vi "GV_LegendVisible.vi"(8 "error in (no error)":errorcluster, 11 "Gviewer in":refnum<class "Gviewer.lvclass">) -> (0 "error out":errorcluster, 1 "Visible?":bool, 3 "Gviewer out":refnum<class "Gviewer.lvclass">)   [LabVIEW 2020, in "Sgraph_lib_V1.lvlib" / "Gviewer.lvclass"]
doc: "Andre Koelewijn, 24 April 2021,\n\nShow/Hide Legend"
uses:
  Gviewer.lvclass
  Gviewer.lvclass/Gviewer.ctl
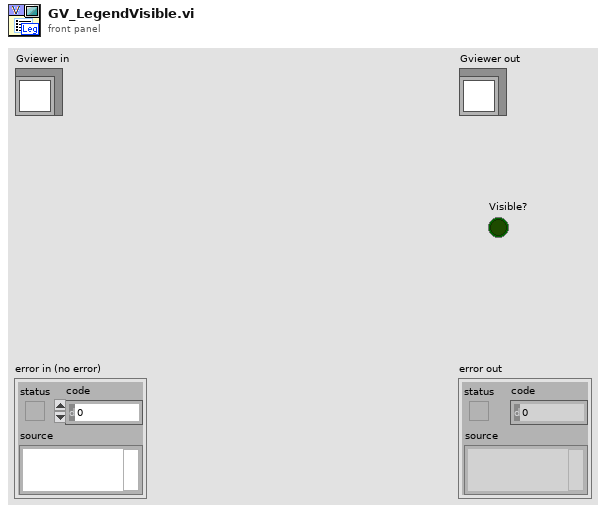
[diagram p1: front panel]
types:
  T1 = typedef "LVPositionTypeDef.ctl" = cluster{"Left":i32, "Top":i32}
  T2 = typedef "LVBoundsTypeDef.ctl" = cluster{"Width":u32, "Height":u32}
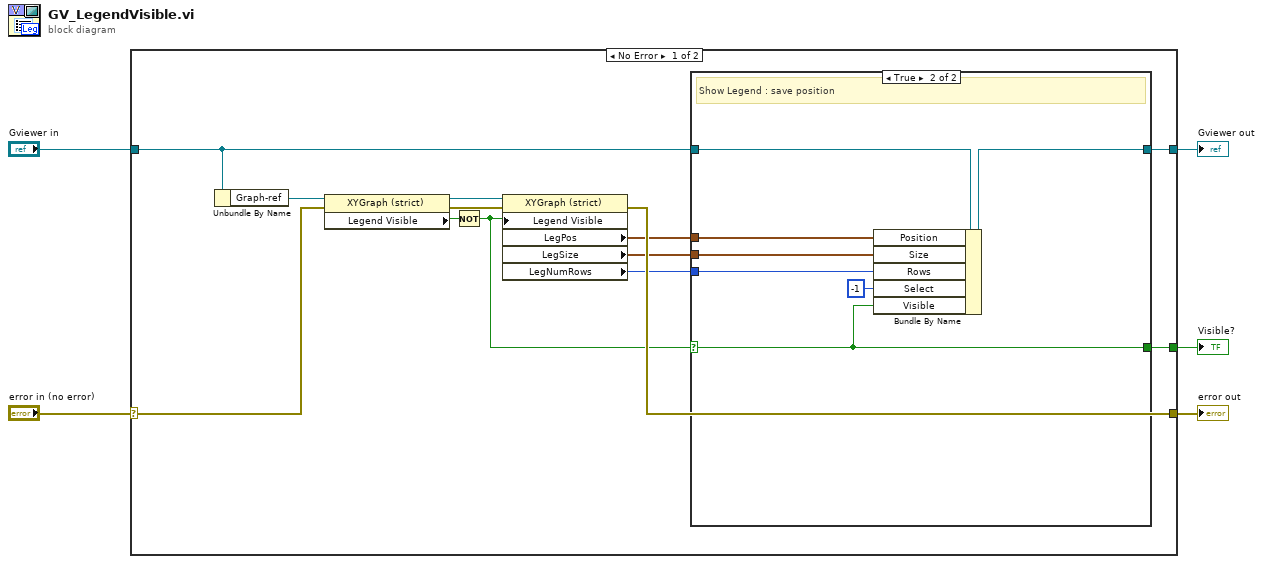
[diagram p0: block diagram]
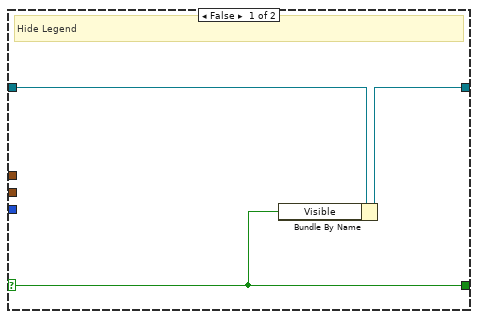
[diagram p2: hidden frame]
diagram:
  n1 = case shown="No Error" "error in (no error)" {
    selector: "error in (no error)" -> [w14 w30]
    tunnel: [w13 w30] -> w4
    tunnel: [w9 w29] -> w2
    tunnel: "Gviewer in" -> [w10 w29]
    tunnel: [w11 _] -> w1
    frame No Error {
      n2 = Unbundle By Name(w10) -> ("Graph-ref"=w15:refnum<vi>)
      n3 = property class="XYGraph (strict)"(reference=w15, error in=w14) -> (reference out=w16:refnum<vi>, error out=w17:errorcluster, "Legend Visible"=w18:bool)
      n4 = Not(x=w18) -> (.not. x?=w12:bool)
      n5 = property class="XYGraph (strict)"(reference=w16, error in=w17, "Legend Visible"=w12) -> (error out=w13:errorcluster, "LegPos"=w8:T1, "LegSize"=w7:T2, "LegNumRows"=w6:u32)  [unwired: 1 out]
      n6 = case shown="True" w12 {
        selector: w12 -> [w21 w22]
        tunnel: [w21 w22] -> w11
        tunnel: w10 -> [w19 w27]
        tunnel: [w20 w28] -> w9
        tunnel: w8 -> [_ w26]
        tunnel: w7 -> [_ w25]
        tunnel: w6 -> [_ w24]
        frame False {
          # "Hide Legend"
          n7 = Bundle By Name(cluster=w19, "Visible"=w21) -> (w20:refnum<class "Gviewer.lvclass">)
        }
        frame True {
          # "Show Legend : save position"
          n8 = Bundle By Name(cluster=w27, "Position"=w26, "Size"=w25, "Rows"=w24, "Select"=-1 ("Legend.Select"), "Visible"=w22) -> (w28:refnum<class "Gviewer.lvclass">)
        }
      }
    }
    frame Error {
    }
  }
  "error out" <- w4
  "Gviewer out" <- w2
  "Visible?" <- w1
